vi "to_json.vi"(8 "error in":errorcluster, 11 "labels in":refnum<class "labels.lvclass">) -> (0 "error out":errorcluster, 2 "json":string, 3 "labels out":refnum<class "labels.lvclass">)   [LabVIEW 2020, in "nominal types.lvlib" / "labels.lvclass"]
uses:
  labels.lvclass
  labels.lvclass/labels.ctl
  b8486177-9344-4009-9026-0c4df4e1a446.vi
  <vilib>/JDP Science/JSONtext/Variant to JSON Text.vi
  <vilib>/JDP Science/JSONtext/LVClass Serializer/JSONtext LVClass Serializer.lvclass
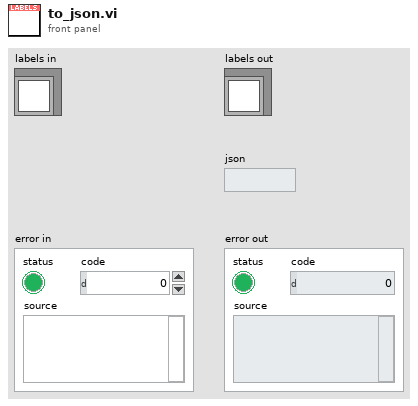
[diagram p1: front panel]
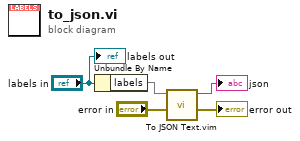
[diagram p0: block diagram]
diagram:
  n1 = Unbundle By Name("labels in") -> ("labels"=w4:set{string})
  n2 = call "To JSON Text.vim"("error in (no error)"="error in", "Anything"=w4) -> ("error out"=→"error out":errorcluster, "<JSON>"=→"json":string)  [unwired: 8 in]
  "labels out" <- "labels in"
